vi "jl stack traces global.vi"() -> ()   [LabVIEW 2018, in "LV2Julia_core.lvlib"]
uses:
  LV2Julia_core.lvlib
  timestamped jl err info.ctl
  detailed error info.ctl
  StackFrame.ctl
panel:
  out "jl exceptions history":T1[](array[typedef]) {"Time Stamp" format="%<%.3X  %x>T"}
  in  "jl exceptions history max items":u32=1024
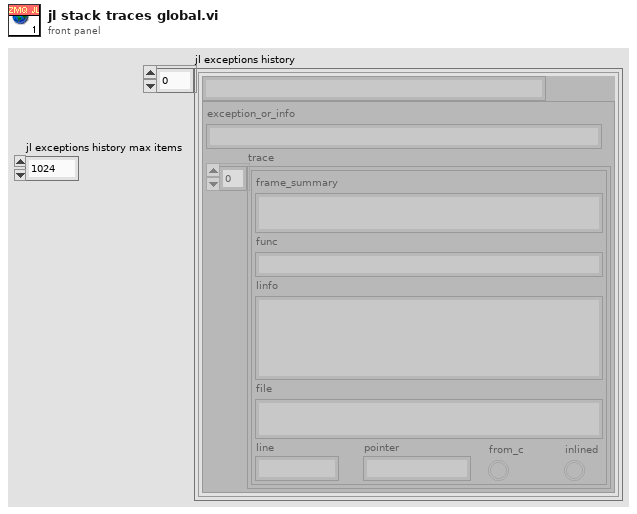
[diagram p1: front panel]
types:
  T1 = typedef "LV2Julia_core.lvlib/timestamped jl err info.ctl" = cluster{"Time Stamp":timestamp, "detailed error info":T2}
  T2 = typedef "LV2Julia_core.lvlib/detailed error info.ctl" = cluster{"exception_or_info":string, "trace":T3[]}
  T3 = typedef "LV2Julia_core.lvlib/StackFrame.ctl" = cluster{"frame_summary":string, "func":string, "linfo":string, "file":string, "line":i32, "pointer":u64, "from_c":bool, "inlined":bool}
diagram:
